vi "Constructor.vi"(0 "Log Instance":refnum<class "LoggerReference.lvclass">, 11 "error in (no error)":errorcluster) -> (4 "class data out":refnum<class "CMESAPI.lvclass">, 15 "error out":errorcluster)   [LabVIEW 2020, in "CMESAPI.lvlib" / "CMESAPI.lvclass"]
uses:
  CMESAPI.lvclass
  <vilib>/gpm_packages/@cs/event-logger/Source/Composed Log/LoggerReference/LoggerReference.lvclass
  D:/Git/Labview-Libraries/Libraries/CMESAPI/CMESAPI_Fw4.0_1.9.2/CMESAPI.dll
  CMESAPI_Fw4.0_1.9.2/CMESAPI.dll
  CMESAPI.lvclass/CMESAPI.ctl
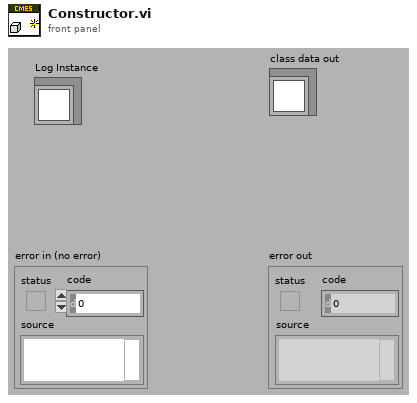
[diagram p1: front panel]
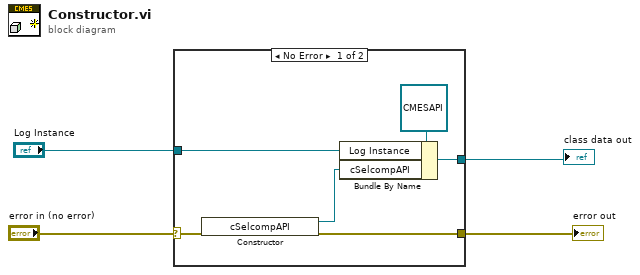
[diagram p0: block diagram]
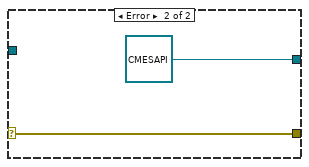
[diagram p2: hidden frame]
diagram:
  n1 = case shown="No Error" "error in (no error)" {
    selector: "error in (no error)" -> [w10 w12]
    tunnel: [w9 w12] -> w3
    tunnel: [w8 refnum<class "CMESAPI.lvclass"> refnum ("class data in")] -> w2
    tunnel: "Log Instance" -> [w7 _]
    frame No Error {
      n2 = constructor class="cSelcompAPI" ("Constructor Node")(error in=w10) -> (reference out=w6:refnum<k24>, error out=w9:errorcluster)  [unwired: 2 in, 1 out]
      n3 = Bundle By Name(cluster=refnum<class "CMESAPI.lvclass"> refnum ("class data in"), "Log Instance"=w7, "cSelcompAPI"=w6) -> (w8:refnum<class "CMESAPI.lvclass">)
    }
    frame Error {
    }
  }
  "error out" <- w3
  "class data out" <- w2
